vi "Get-position-profile.vi"(8 "error in (no error)":errorcluster, 11 "Motor-Maxon in":refnum<class "Motor-Maxon.lvclass">) -> (0 "error out":errorcluster, 2 "Position profile":T1, 3 "Motor-Maxon out":refnum<class "Motor-Maxon.lvclass">)   [LabVIEW 2013, in "PowderDeposition.lvlib" / "Motor-Maxon.lvclass"]
uses:
  Motor-Maxon.lvclass
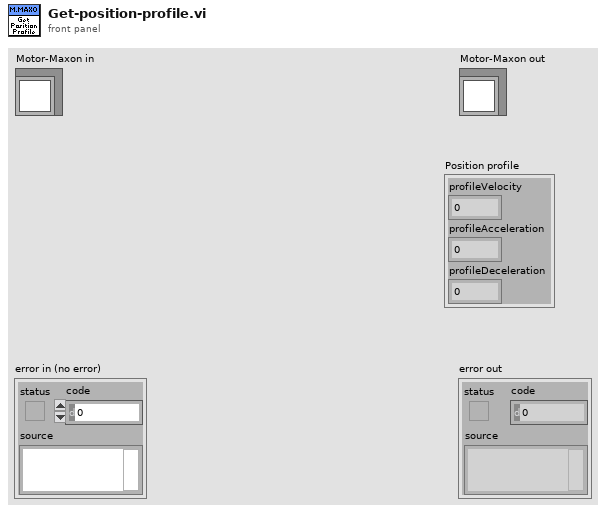
[diagram p1: front panel]
types:
  T1 = cluster{"profileVelocity":u32, "profileAcceleration":u32, "profileDeceleration":u32}
  T2 = typedef "PowderDeposition.lvlib/Motor.lvclass/Action-settings.ctl" = cluster{"Speed":dbl, "Acceleration":dbl, "Direction":enum16{"Clockwise", "Counter-clockwise"}}
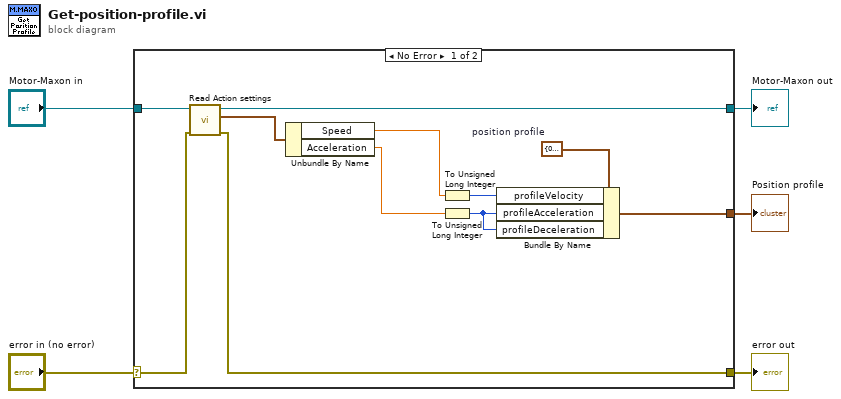
[diagram p0: block diagram]
diagram:
  n1 = case shown="No Error" "error in (no error)" {
    selector: "error in (no error)" -> [w8 w18]
    tunnel: [w7 w18] -> w4
    tunnel: [w15 w17] -> w2
    tunnel: "Motor-Maxon in" -> [w16 w17]
    tunnel: [w6 _] -> w1
    frame No Error {
      w13 = T1 {"profileVelocity"=0, "profileAcceleration"=0, "profileDeceleration"=0}  # position profile
      n2 = call-dynamic "Read Action settings.vi"("error in (no error)"=w8, "Motor in"=w16) -> ("error out"=w7:errorcluster, "Action settings"=w14:T2, "Motor out"=w15:refnum<class "Motor-Maxon.lvclass">)  [unwired: 7 in]
      n3 = Unbundle By Name(w14) -> ("Speed"=w12:dbl, "Acceleration"=w10:dbl)
      n4 = To Unsigned Long Integer(number=w12) -> (unsigned 32bit integer=w11:u32)
      n5 = To Unsigned Long Integer(number=w10) -> (unsigned 32bit integer=w9:u32)
      n6 = Bundle By Name(cluster=w13, "profileVelocity"=w11, "profileAcceleration"=w9, "profileDeceleration"=w9) -> (w6:T1)
    }
    frame Error {
    }
  }
  "error out" <- w4
  "Motor-Maxon out" <- w2
  "Position profile" <- w1
